vi "executeSequenceFile.vi"(8 "EntryPoint":string, 9 "ProcessModelPath":string, 10 "sequenceFile":refnum<k7>, 11 "Sequence Context In":refnum<k7>) -> (0 "error out":errorcluster)   [LabVIEW 2011]
doc: "Executes the specified process model entry point, using the specified sequence file as the client sequence file."
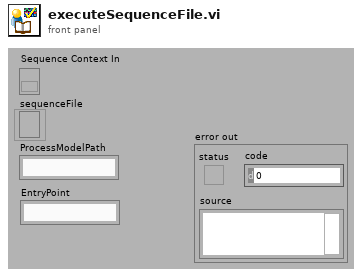
[diagram p1: front panel]
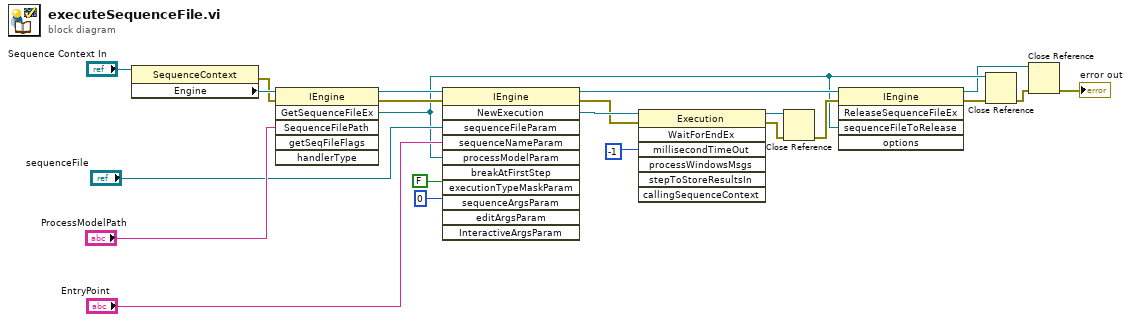
[diagram p0: block diagram]
diagram:
  n1 = property class="SequenceContext"(reference="Sequence Context In") -> (error out=w3:errorcluster, "Engine"=w20:refnum<k7>)  [unwired: 1 in, 1 out]
  n2 = invoke class="IEngine" method="GetSequenceFileEx"(reference=w20, error in=w3, "SequenceFilePath"="ProcessModelPath") -> (reference out=w19:refnum<k7>, error out=w18:errorcluster, "GetSequenceFileEx"=w7:refnum<k7>)  [unwired: 3 in, 3 out]
  n3 = invoke class="IEngine" method="NewExecution"(reference=w19, error in=w18, "sequenceFileParam"="sequenceFile", "sequenceNameParam"="EntryPoint", "processModelParam"=w7, "breakAtFirstStep"=FALSE, "executionTypeMaskParam"=0) -> (reference out=w10:refnum<k7>, error out=w14:errorcluster, "NewExecution"=w15:refnum<k7>)  [unwired: 4 in, 8 out]
  n4 = invoke class="Execution" method="WaitForEndEx"(reference=w15, error in=w14, "millisecondTimeOut"=-1) -> (reference out=w11:refnum<k7>, error out=w12:errorcluster)  [unwired: 4 in, 5 out]
  n5 = Close Reference(reference=w11, error in (no error)=w12) -> (error out=w9:errorcluster)
  n6 = invoke class="IEngine" method="ReleaseSequenceFileEx"(reference=w10, error in=w9, "sequenceFileToRelease"=w7) -> (reference out=w5:refnum<k7>, error out=w8:errorcluster)  [unwired: 2 in, 3 out]
  n7 = Close Reference(reference=w7, error in (no error)=w8) -> (error out=w6:errorcluster)
  n8 = Close Reference(reference=w5, error in (no error)=w6) -> (error out=→"error out":errorcluster)
